vi "UDP Named Service - ANC Rotator Server.vi"() -> ()   [LabVIEW 2025]
doc: "Creates a named service and listens on the first available port. When a client connects to the service, it sends a response string to the client.\nAuthor: Scott Hannahs <sth@magnet.fsu.edu>\n\nThis software is licensed for use under the “MIT License\"\nCopyright (c) 2025 Scott Hannahs, sth@sth@magnet.sthnet.net\n\nPermission is hereby granted, free of charge, to any person obtaining a copy of this software and associated documentation files (the \"Software\"), to deal in the Software without restriction, including without limitation the rights to use, copy, modify, merge, publish, distribute, sublicense, and/or sell copies of the Software, and to permit persons to whom the Software is furnished to do so, subject to the following conditions: The above copyright notice and this permission notice shall be included in all copies or substantial portions of the Software.\n\nTHE SOFTWARE IS PROVIDED \"AS IS\", WITHOUT WARRANTY OF ANY KIND, EXPRESS OR IMPLIED, INCLUDING BUT NOT LIMITED TO THE WARRANTIES OF MERCHANTABILITY, FITNESS FOR A PARTICULAR PURPOSE AND NONINFRINGEMENT. IN NO EVENT SHALL THE AUTHORS OR COPYRIGHT HOLDERS BE LIABLE FOR ANY CLAIM, DAMAGES OR OTHER LIABILITY, WHETHER IN AN ACTION OF CONTRACT, TORT OR OTHERWISE, ARISING FROM, OUT OF OR IN CONNECTION WITH THE SOFTWARE OR THE USE OR OTHER DEALINGS IN THE SOFTWARE."
uses:
  <vilib>/Utility/error.llb/Trim Whitespace One-Sided.vi
panel:
  out "Port":u16
  out "Status String":string
  in  "Stop":bool
  # "Overview: Demonstrates the use of the UDP functions to initialize a named UDP service that can send data to a client VI.\nInstructions:\n1. Run the VI.\n2. Open UDP Named Service - Client.vi and follow the instructions on its front panel.\n3. Click Stop to stop the VI."
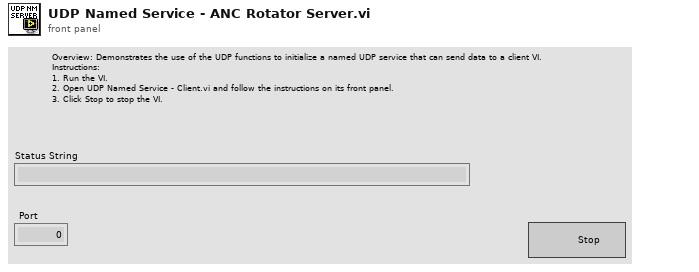
[diagram p1: front panel]
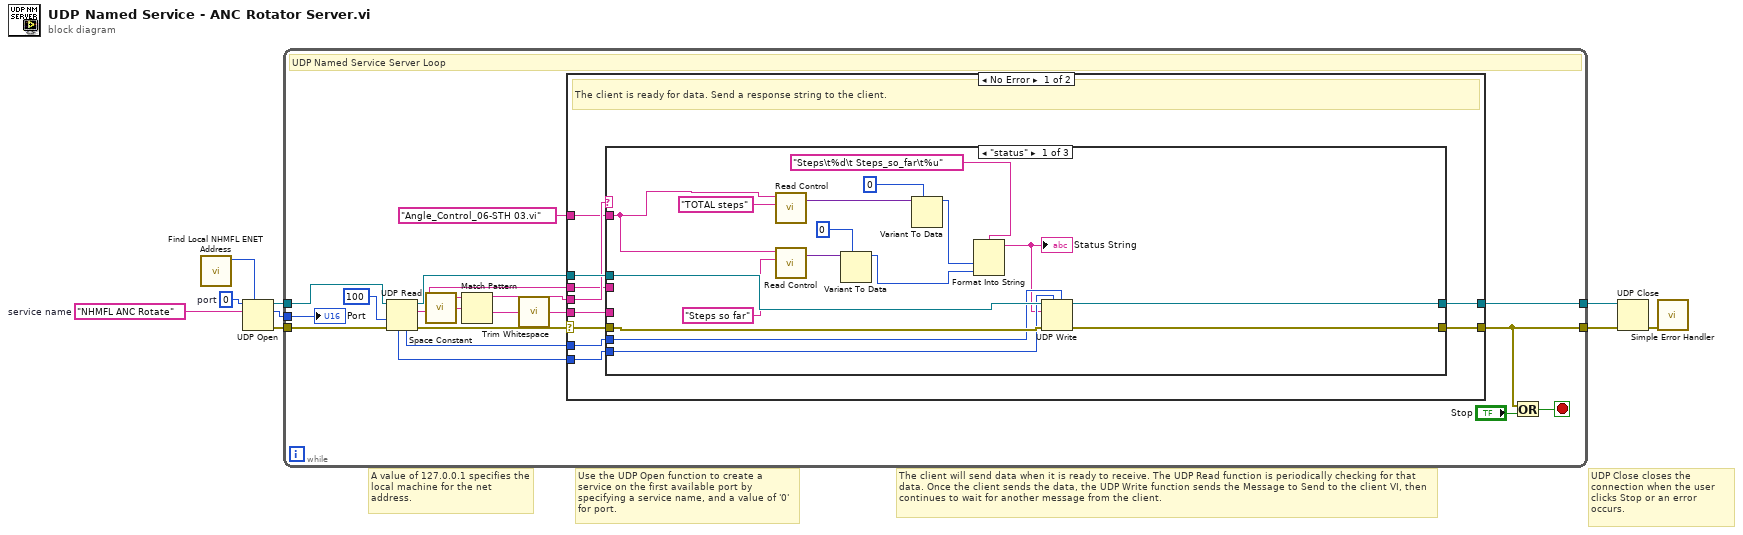
[diagram p0: block diagram]
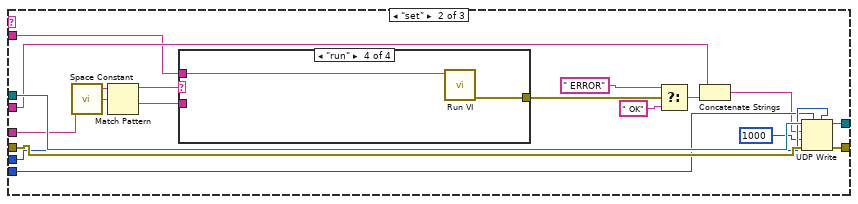
[diagram p2: hidden frame]
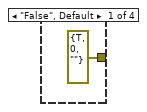
[diagram p3: hidden frame]
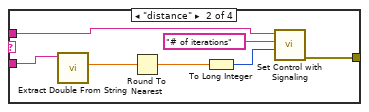
[diagram p4: hidden frame]
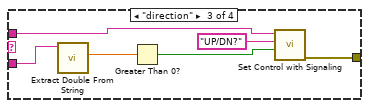
[diagram p5: hidden frame]
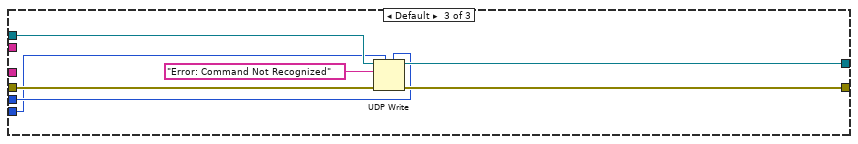
[diagram p6: hidden frame]
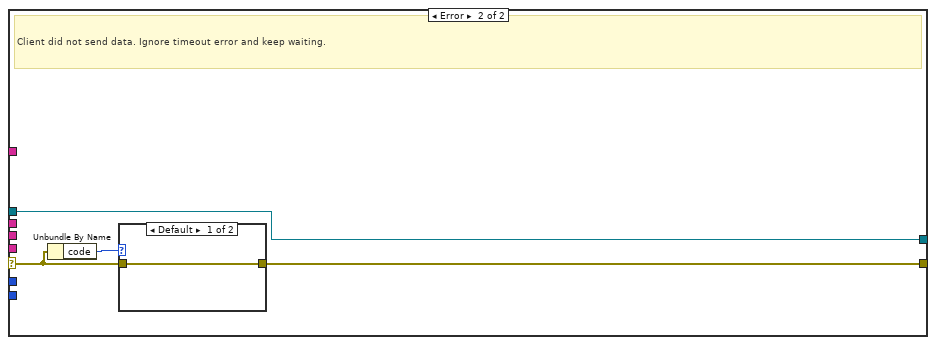
[diagram p7: hidden frame]
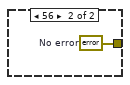
[diagram p8: hidden frame]
diagram:
  w2 = u16 0  # port
  w9 = "NHMFL ANC Rotate"  # service name
  # "UDP Close closes the connection when the user clicks Stop or an error occurs."
  # "A value of 127.0.0.1 specifies the local machine for the net address."
  # "The client will send data when it is ready to receive. The UDP Read function is periodically checking for that data. Once the client sends the data, the UDP Write function sends the Message to Send to the client VI, then continues to wait for another message from the client."
  # "Use the UDP Open function to create a service on the first available port by specifying a service name, and a value of '0' for port."
  n1 = call "Find Local NHMFL ENET Address.vi"() -> ("Ethernet Address"=w1:u32)  [unwired: 9 in, 2 out]
  n2 = UDP Open(7:w1, 10:w9, 11:w2) -> (port=w8:refnum<k16>, 0:w7:errorcluster, 2:w4:u16)  [unwired: 2 in]
  n3 = while {
    tunnel: [w18] -> w5
    tunnel: w8 -> [w27]
    tunnel: w7 -> [w23]
    tunnel: [w24] -> w6
    tunnel: w4 -> [w21]
    stop <- w20 stop-if-true
    # "UDP Named Service Server Loop"
    n4 = UDP Read(connection ID=w27, timeout ms (25000)=100, 8:w23) -> (data out=w11:string, error out=w26:errorcluster, 3:w25:refnum<k16>, 4:w22:u16, 6:w16:u32)  [unwired: 1 in]
    n5 = call <vilib>:"Space Constant.vi"() -> ("String"=w12:string)
    n6 = Match Pattern(string=w11, regular expression=w12) -> (before substring=w15:string, after substring=w14:string)  [unwired: 1 in, 2 out]
    n7 = call <vilib>:"Trim Whitespace.vi"("string"=w14) -> ("trimmed string"=w13:string)  [unwired: 1 in]
    n8 = case shown="No Error" w26 {
      selector: w26 -> [w37 w98]
      tunnel: w25 -> [w34 w99]
      tunnel: [w36 w96] -> w18
      tunnel: [w35 w99] -> w24
      tunnel: w16 -> [w32 _]
      tunnel: w22 -> [w33 _]
      tunnel: w15 -> [w31 _]
      tunnel: w13 -> [w30 _]
      tunnel: w11 -> [w29 _]
      tunnel: "Angle_Control_06-STH 03.vi" -> [w28 _]
      frame No Error {
        # "The client is ready for data. Send a response string to the client."
        n9 = case shown="\"status\"" w31 {
          tunnel: w37 -> [w54 w72 w95]
          tunnel: [w53 w71 w94] -> w36
          tunnel: [w52 w70 w93] -> w35
          tunnel: w34 -> [w51 w69 w92]
          tunnel: w33 -> [w50 w68 w91]
          tunnel: w32 -> [w49 w67 w90]
          tunnel: w30 -> [_ w66 _]
          tunnel: w29 -> [_ w62 _]
          tunnel: w28 -> [w42 w55 _]
          frame "status" {
            n10 = call "Read Control.vi"("VI Name"=w42, "Control Name"="TOTAL steps") -> ("Value"=w47:variant)  [unwired: 3 in, 1 out]
            n11 = call "Read Control.vi"("VI Name"=w42, "Control Name"="Steps so far") -> ("Value"=w40:variant)  [unwired: 3 in, 1 out]
            n12 = Variant To Data(type=u32 0, Variant=w40) -> (data=w38:u32)  [unwired: 1 in, 1 out]
            n13 = Variant To Data(type=0, Variant=w47) -> (data=w45:i32)  [unwired: 1 in, 1 out]
            n14 = Format Into String(format string="Steps\t%d\t Steps_so_far\t%u", w45, w38) -> (resulting string=w43:string)  [unwired: 2 in, 1 out]
            "Status String" <- w43
            n15 = UDP Write(address=w49, port or service name=w50, connection ID=w51, data in=w43, 8:w54) -> (error out=w53:errorcluster, 3:w52:refnum<k16>)  [unwired: 1 in]
          }
          frame "set" {
            n16 = call <vilib>:"Space Constant.vi"() -> ("String"=w65:string)
            n17 = Match Pattern(string=w66, regular expression=w65) -> (before substring=w64:string, after substring=w63:string)  [unwired: 1 in, 2 out]
            n18 = case shown="\"run\"" w64 {
              tunnel: w63 -> [_ w77 w83 _]
              tunnel: w55 -> [_ w79 w85 w88]
              tunnel: [errorcluster {"status"=TRUE, "code"=0, "source"=""} ("error out") w76 w82 w87] -> w61
              frame "False", Default {
              }
              frame "distance" {
                n19 = call "Extract Double From String.vi"("string"=w77) -> ("floating pt. number"=w78:dbl)  [unwired: 3 in, 3 out]
                n20 = Round To Nearest(number=w78) -> (nearest integer value=w75:dbl)
                n21 = To Long Integer(number=w75) -> (32bit integer=w74:i32)
                n22 = call "Set Control with Signaling.vi"("Value"=w74, "Control Name"="# of iterations", "VI Name"=w79) -> ("error out"=w76:errorcluster)  [unwired: 8 in]
              }
              frame "direction" {
                n23 = call "Extract Double From String.vi"("string"=w83) -> ("floating pt. number"=w84:dbl)  [unwired: 3 in, 3 out]
                n24 = Greater Than 0?(x=w84) -> (x > 0?=w81:bool)
                n25 = call "Set Control with Signaling.vi"("Value"=w81, "Control Name"="UP/DN?", "VI Name"=w85) -> ("error out"=w82:errorcluster)  [unwired: 8 in]
              }
              frame "run" {
                n26 = call "Run VI.vi"("VI Name"=w88) -> ("error out"=w87:errorcluster)  [unwired: 10 in]
              }
            }
            n27 = Select(t=" ERROR", s=w61, f=" OK") -> (s? t:f=w57:string)
            n28 = Concatenate Strings(w62, w57) -> (w56:string)
            n29 = UDP Write(address=w67, port or service name=w68, connection ID=w69, data in=w56, 8:w72, 9:1000 ("timeout ms (25000)")) -> (error out=w71:errorcluster, 3:w70:refnum<k16>)
          }
          frame Default {
            n30 = UDP Write(address=w90, port or service name=w91, connection ID=w92, data in="Error: Command Not Recognized", 8:w95) -> (error out=w94:errorcluster, 3:w93:refnum<k16>)  [unwired: 1 in]
          }
        }
      }
      frame Error {
        # "Client did not send data. Ignore timeout error and keep waiting."
        n31 = Unbundle By Name(w98) -> ("code"=w97:i32)
        n32 = case shown="Default" w97 {
          tunnel: w98 -> [w100 _]
          tunnel: [w100 w101] -> w96
          frame Default {
          }
          frame 56 {
            w101 = errorcluster {"status"=FALSE, "code"=0, "source"=""}  # No error
          }
        }
      }
    }
    n33 = Or(x=w18, y="Stop") -> (x .or. y?=w20:bool)
    "Port" <- w21
  }
  n34 = UDP Close(connection ID=w6, 8:w5) -> (error out=w3:errorcluster)  [unwired: 1 out]
  n35 = call <vilib>:"Simple Error Handler.vi"("error in (no error)"=w3) -> ()  [unwired: 4 in, 5 out]
